vi "Enqueue Element.vi"(6 "Priority? (F)":bool, 8 "error in":errorcluster, 9 "Data":variant, 10 "State":T1=enum."Start timer") -> (0 "error out":errorcluster)   [LabVIEW 2018, in "Covers-o-meter.lvlib"]
doc: "Enqueues element"
uses:
  Covers-o-meter.lvlib
  ctl/State--enum.ctl
  ctl/Queue action--enum.ctl
  ctl/Message--enum.ctl
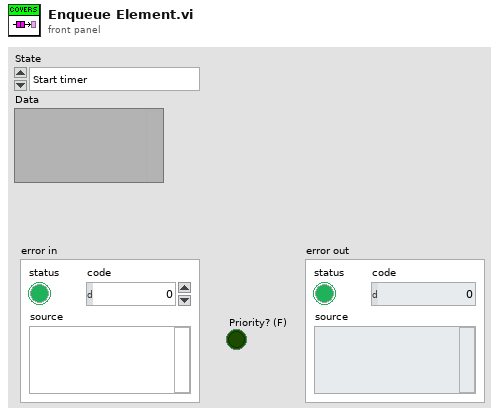
[diagram p1: front panel]
types:
  T1 = typedef "Covers-o-meter.lvlib/State--enum.ctl" = enum16{"Init", "Init: Read req tags", "Init Data: All Projects", "Init: Which Project?", "Update Requirements tags", "Get all project strings", "Search proj for tags", "Subroutine", "Update Project", "Start Button Pressed", "Start timer", "Error", "Close", "UI - Refresh Timer ", "UI - refresh graph", "UI - Refresh Tree"}
  T2 = typedef "Covers-o-meter.lvlib/Message--enum.ctl" = cluster{"State":T1, "Data":variant}
  T3 = typedef "Covers-o-meter.lvlib/Queue action--enum.ctl" = enum16{"Create", "Get", "Destroy"}
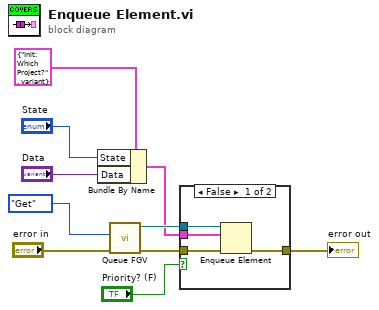
[diagram p0: block diagram]
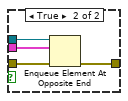
[diagram p2: hidden frame]
diagram:
  n1 = Bundle By Name(cluster=T2 {"State"=enum."Init: Which Project?", "Data"=variant} ("Message"), "State"="State", "Data"="Data") -> (w1:T2)
  n2 = call "Queue FGV.vi"("error in"="error in", "Queue Action"=Queue_action--enum."Get") -> ("error out"=w6:errorcluster, "Queue reference"=w7:refnum<queue>)  [unwired: 8 in]
  n3 = case shown="False" "Priority? (F)" {
    tunnel: [w14 w18] -> w9
    tunnel: w7 -> [w13 w17]
    tunnel: w6 -> [w12 w15]
    tunnel: w1 -> [w11 w16]
    frame False {
      n4 = Enqueue Element(queue=w13, element=w11, error in (no error)=w12) -> (error out=w14:errorcluster)  [unwired: 1 in, 2 out]
    }
    frame True {
      n5 = Enqueue Element At Opposite End(queue=w17, element=w16, error in (no error)=w15) -> (error out=w18:errorcluster)  [unwired: 1 in, 2 out]
    }
  }
  "error out" <- w9
